vi "CLD 4 Event Structure Timer Solution.vi"() -> ()   [LabVIEW 2019]
doc: "CLD 4 Challenge Exercise\n\nThis VI demonstrates the use of the time out constant for the event structure in conjunction with some processing of values.\n\nAlthough the front panel behaves similar to the timers in previous CLD exercises, it is not reliable as a time tracking device. The timing only counts the number of time outs, and associates a time with each occurrence of the time out.\n\nIf there were to be any other events that occur, then the timing would not be consecutive time. Using the time out functionality of an event structure for actual process timing is not a viable method, unless inactivity is being timed."
panel:
  out "Elapsed Time":dbl
  out "Error Out":errorcluster
  in  "Error In":errorcluster
  out "Bit 4":bool
  out "Bit 3":bool
  out "Bit 2":bool
  out "Bit 1":bool
  out "Time Has Elapsed":bool
  in  "Auto Reset":bool=TRUE
  in  "Reset Button":bool
  in  "Stop VI":bool
  in  "Time Target (s)":dbl=4.0
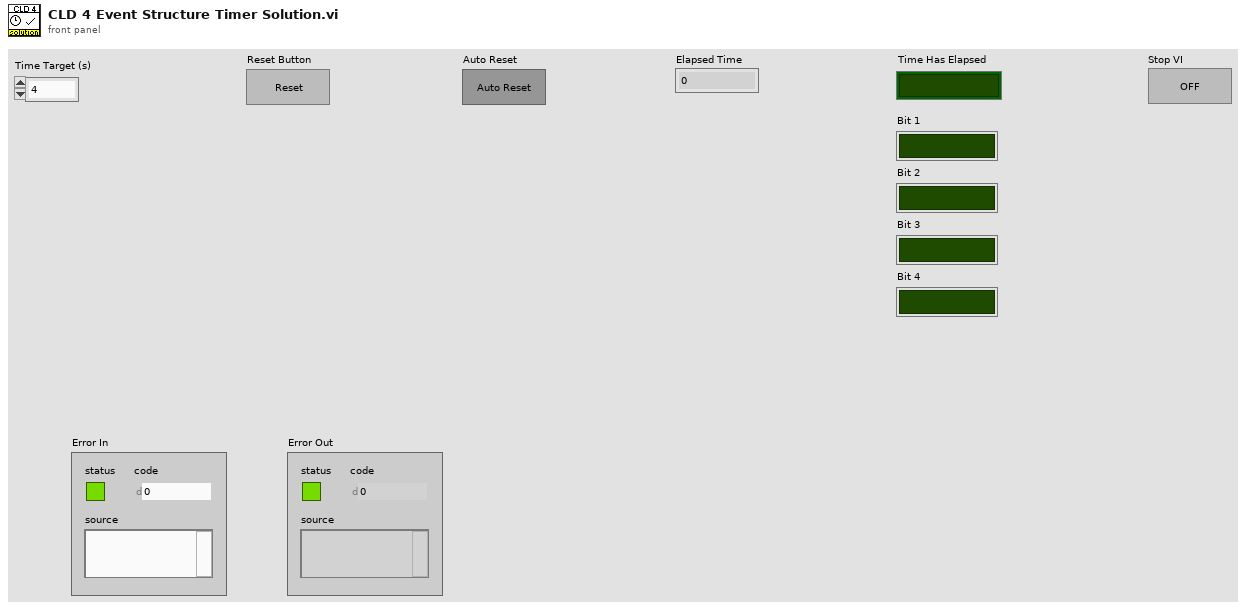
[diagram p1: front panel]
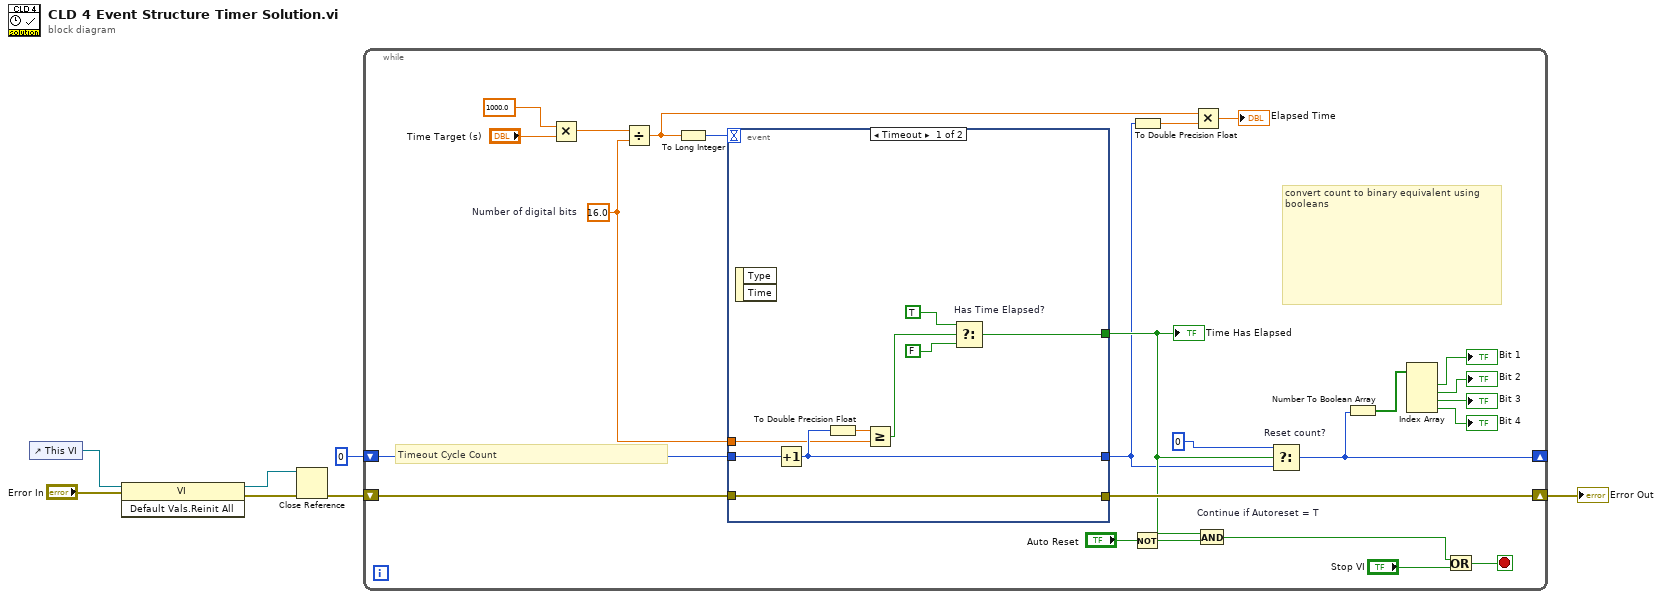
[diagram p0: block diagram]
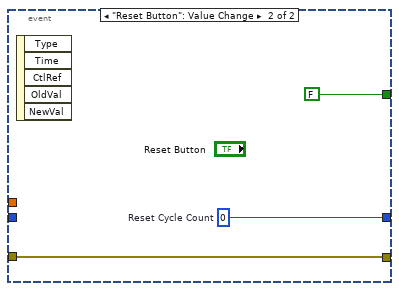
[diagram p2: hidden frame]
diagram:
  n1 = control-ref of="This VI"() -> (w3:refnum<vi>)
  n2 = invoke class="VI" method="Default Vals.Reinit All"(reference=w3, error in="Error In") -> (reference out=w1:refnum<vi>, error out=w4:errorcluster)  [unwired: 1 in, 1 out]
  n3 = Close Reference(reference=w1, error in (no error)=w4) -> (error out=w2:errorcluster)
  n4 = while {
    shift-right: [w12] -> _
    shift-left: 0 -> [w31]
    shift-right: [w24] -> w5
    shift-left: w2 -> [w25]
    stop <- w20 stop-if-true
    w11 = 16.0  # Number of digital bits
    # "convert count to binary equivalent using booleans"
    # "Timeout Cycle Count"
    n5 = Multiply(x=1000.0, y="Time Target (s)") -> (x*y=w22:dbl)
    n6 = Divide(x=w22, y=w11) -> (x/y=w18:dbl)
    n7 = To Long Integer(number=w18) -> (32bit integer=w8:i32)
    n8 = event shown="[0] Timeout" {
      selector: _ -> [_ _]
      dyn-events: _ -> [_ _]
      timeout: w8 -> [_ _]
      tunnel: [w35 w43] -> w13
      tunnel: w31 -> [w41 _]
      tunnel: [w37 FALSE] -> w15
      tunnel: w25 -> [w36 w42]
      tunnel: [w36 w42] -> w24
      tunnel: w11 -> [w34 _]
      event Timeout {
        n9 = event-data() -> ()  [unwired: 1 in, 2 out]
        n10 = Increment(x=w41) -> (x+1=w35:i32)
        n11 = To Double Precision Float(number=w35) -> (double precision float=w33:dbl)
        n12 = Greater Or Equal?(x=w33, y=w34) -> (x >= y?=w40:bool)
        n13 = Select "Has Time Elapsed?"(t=TRUE, s=w40, f=FALSE) -> (s? t:f=w37:bool)
      }
      event "Reset Button": Value Change {
        w43 = 0  # Reset Cycle Count
        n14 = event-data() -> ()  [unwired: 1 in, 5 out]
      }
    }
    "Time Has Elapsed" <- w15
    n15 = Not(x="Auto Reset") -> (.not. x?=w16:bool)
    n16 = To Double Precision Float(number=w13) -> (double precision float=w10:dbl)
    n17 = Multiply(x=w18, y=w10) -> (x*y=→"Elapsed Time":dbl)
    n18 = And "Continue if Autoreset = T"(x=w15, y=w16) -> (x .and. y?=w19:bool)
    n19 = Select "Reset count?"(t=0, s=w15, f=w13) -> (s? t:f=w12:i32)
    n20 = Number To Boolean Array(number=w12) -> (Boolean array=w30:bool[])
    n21 = Index Array(array=w30) -> (element #1=→"Bit 1":bool, element #2=→"Bit 2":bool, element #3=→"Bit 3":bool, element #4=→"Bit 4":bool)  [unwired: 4 in]
    n22 = Or(x=w19, y="Stop VI") -> (x .or. y?=w20:bool)
  }
  "Error Out" <- w5
